vi "file_read_size.vi"(8 "error in (no error)":errorcluster, 11 "filepath":path) -> (0 "error out":errorcluster, 2 "size_bytes":i64)   [LabVIEW 2015, in "lv-dropbox.lvlib" / "v2.lvlib"]
uses:
  v2.lvlib
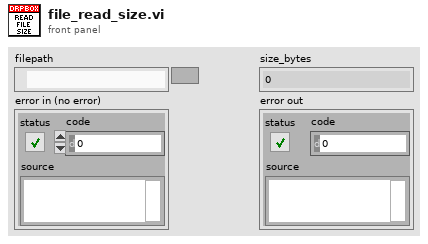
[diagram p1: front panel]
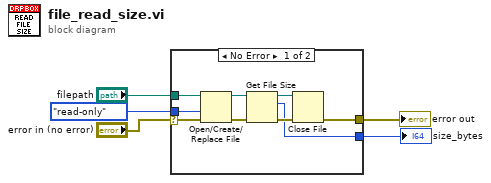
[diagram p0: block diagram]
diagram:
  n1 = case shown="No Error" "error in (no error)" {
    selector: "error in (no error)" -> [w8 w15]
    tunnel: enum16{"read/write", "read-only", "write-only"}."read-only" ("access (0:read/write)") -> [w14 _]
    tunnel: [w12 _] -> w4
    tunnel: "filepath" -> [w9 _]
    tunnel: [w7 w15] -> w1
    frame No Error {
      n2 = Open/Create/Replace File(file path (use dialog)=w9, error in=w8, access (0:read/write)=w14) -> (refnum out=w10:refnum<file>, error out=w11:errorcluster)  [unwired: 3 in, 1 out]
      n3 = Get File Size(file=w10, error in=w11) -> (refnum out=w6:refnum<file>, size (in bytes)=w12:i64, 0:w13:errorcluster)
      n4 = Close File(refnum=w6, error in=w13) -> (error out=w7:errorcluster)  [unwired: 1 out]
    }
    frame Error {
    }
  }
  "error out" <- w1
  "size_bytes" <- w4
